vi "Initialise.vi"(8 "error in (no error)":errorcluster, 10 "Instrument Ref":string, 11 "Hioki BT4560B in":refnum<class "Hioki BT4560B.lvclass">) -> (0 "error out":errorcluster, 3 "Hioki BT4560B out":refnum<class "Hioki BT4560B.lvclass">)   [LabVIEW 2021, in "Concrete.lvlib" / "Hioki BT4560B.lvclass"]
uses:
  Hioki BT4560B.lvclass
  Hioki BT4560B.lvclass/Hioki BT4560B.ctl
  Harware Abstraction/AnalogIO/AIO.lvclass
  <instrlib>/HIOKI BT4560/HIOKI BT4560.lvlib
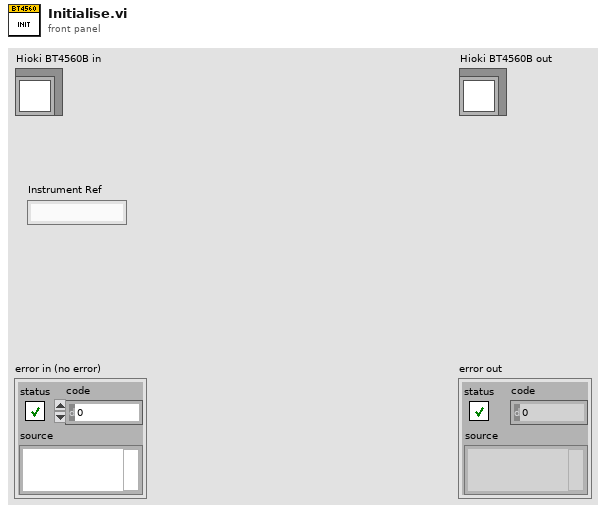
[diagram p1: front panel]
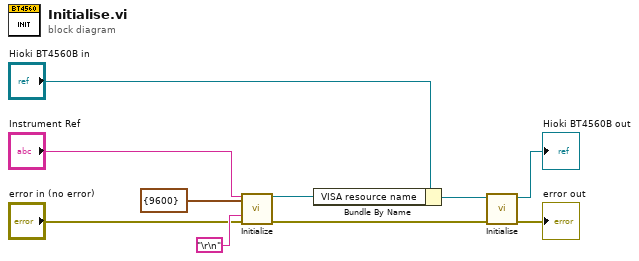
[diagram p0: block diagram]
diagram:
  n1 = call <instrlib>:"Initialize.vi"("VISA resource name"="Instrument Ref", "Serial Configuration"=cluster{"Baud Rate":u32} {"Baud Rate"=9600} ("Configuration"), "Terminator"="\r\n", "error in (no error)"="error in (no error)") -> ("VISA resource name out"=w2:refnum<visa-resource-name>, "error out"=w6:errorcluster)  [unwired: 9 in, 1 out]
  n2 = Bundle By Name(cluster="Hioki BT4560B in", "VISA resource name"=w2) -> (w1:refnum<class "Hioki BT4560B.lvclass">)
  n3 = call-parent "Initialise.vi"("error in (no error)"=w6, "Instrument in"=w1) -> ("error out"=→"error out":errorcluster, "Instrument out"=→"Hioki BT4560B out":refnum<class "Hioki BT4560B.lvclass">)  [unwired: 8 in]
